vi "FunctionSolverQuadratic.vi"(0 "a":dbl, 1 "b":dbl, 2 "c":dbl, 3 "d":dbl, 4 "x":dbl) -> (5 "f(x)":dbl)   [LabVIEW 2021]
doc: "Takes x value and coefficients of a quadratic function on form f(x) = ax²+bx+c+d and returns the result."
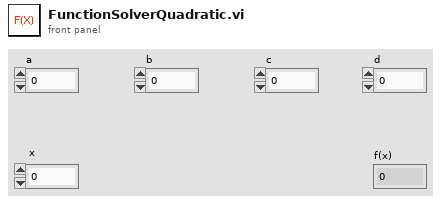
[diagram p1: front panel]
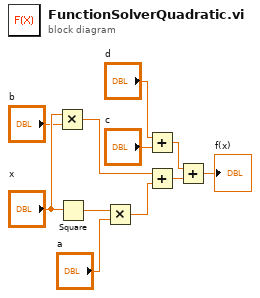
[diagram p0: block diagram]
diagram:
  n1 = Multiply(x="x", y="b") -> (x*y=w6:dbl)
  n2 = Square(x="x") -> (x^2=w10:dbl)
  n3 = Multiply(x=w10, y="a") -> (x*y=w9:dbl)
  n4 = Add(x="d", y="c") -> (x+y=w3:dbl)
  n5 = Add(x=w6, y=w9) -> (x+y=w2:dbl)
  n6 = Add(x=w3, y=w2) -> (x+y=→"f(x)":dbl)
